vi "Add_Part_of_Track(101_and_11)-1.vi"(0 "[IN] Still connected\ntracks in group":T2, 1 "[IN] i for Probl\nem  Point Index":i32, 2 "[IN] i for # of Track \nwith Problem Point":i32, 3 "[IN] Minimal Sub\ntrack Length":i32, 7 "[IN] Subtrack":T1, 9 "[IN] Index in subtrack":i32, 11 "error IN":errorcluster, 12 "[IN] Index of problem\npoint inside subtrack":i32, 13 "[IN] # of subtrack conta\nining problem point":i32) -> (8 "[OUT] Subtrack":T1, 10 "[OUT] Last point in subtrack":i32, 15 "error OUT":errorcluster)   [LabVIEW 2013]
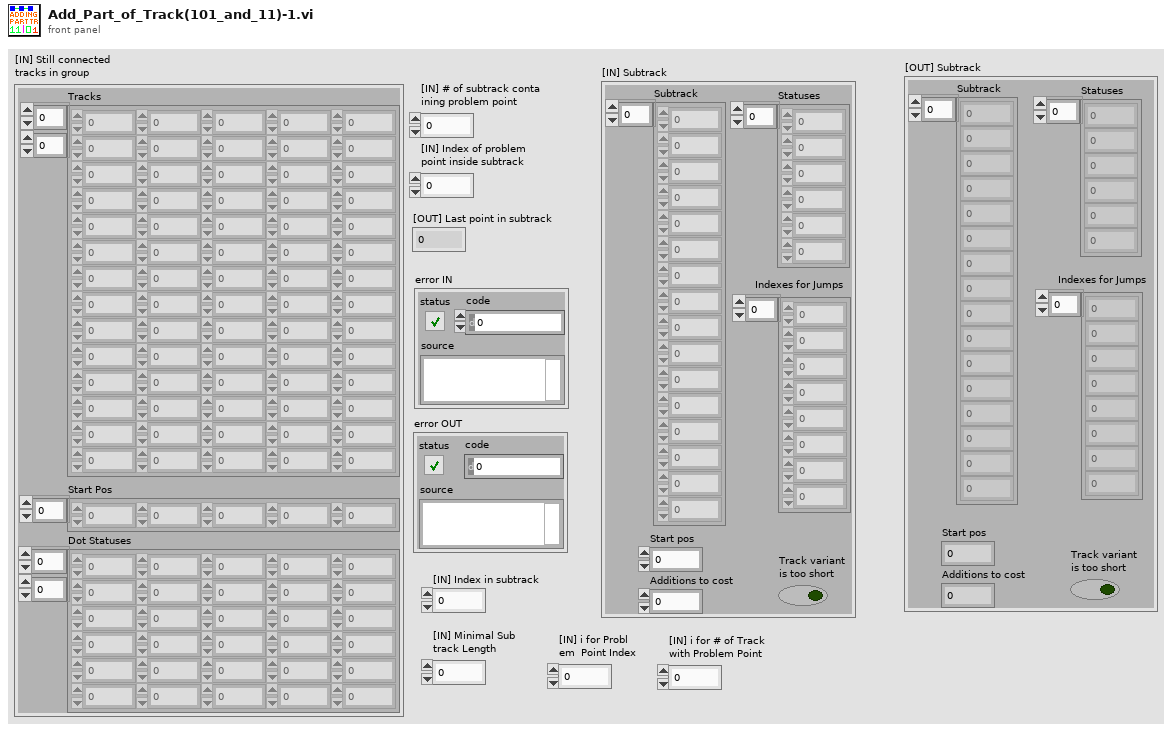
[diagram p1: front panel]
types:
  T1 = cluster{"Subtrack":dbl[], "Statuses":i16[], "Start pos":i32, "Additions to cost":i32, "Track variant \nis too short":bool, "Indexes for Jumps":i32[]}
  T2 = cluster{"Tracks":dbl[][], "Start Pos":i32[], "Dot Statuses":i16[][]}
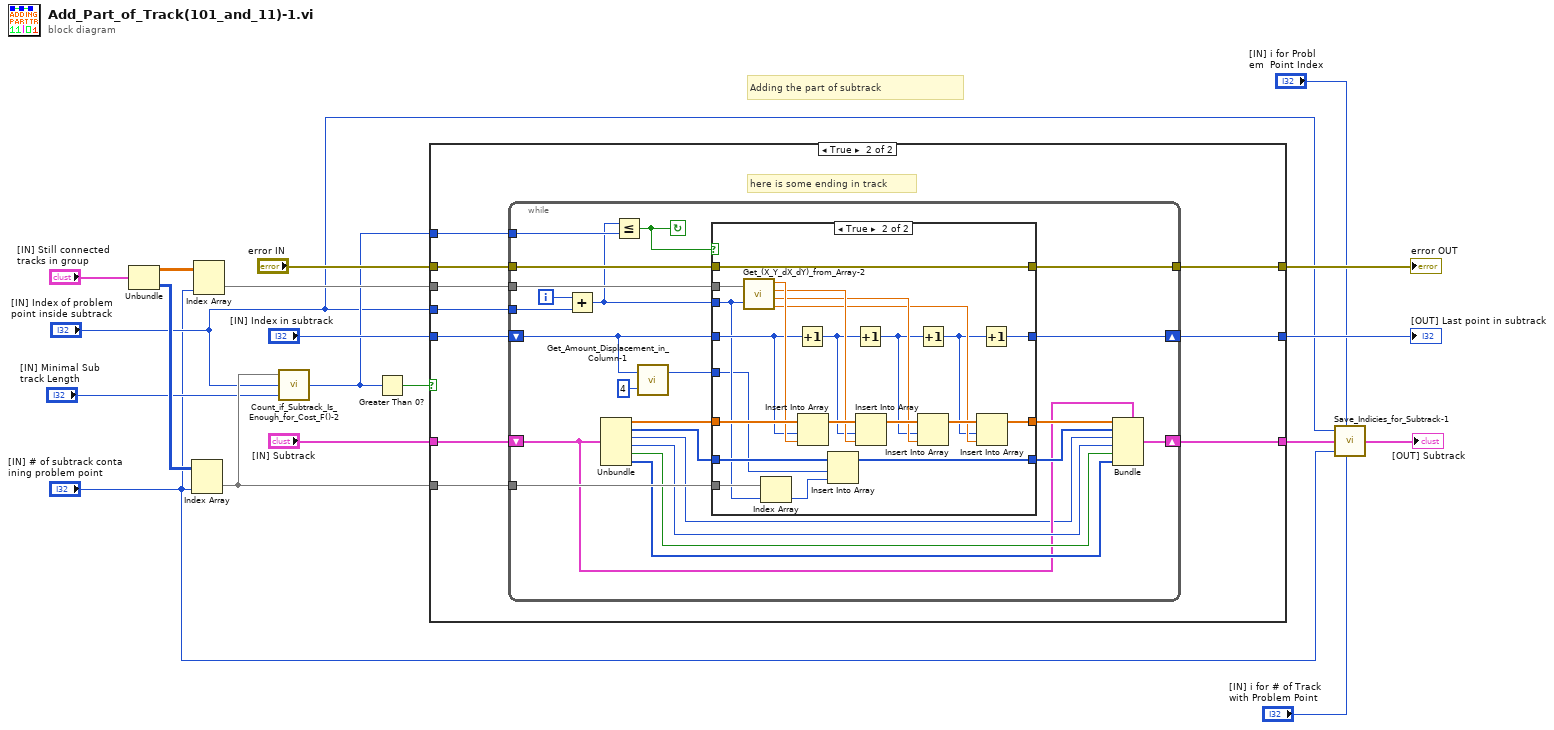
[diagram p0: block diagram]
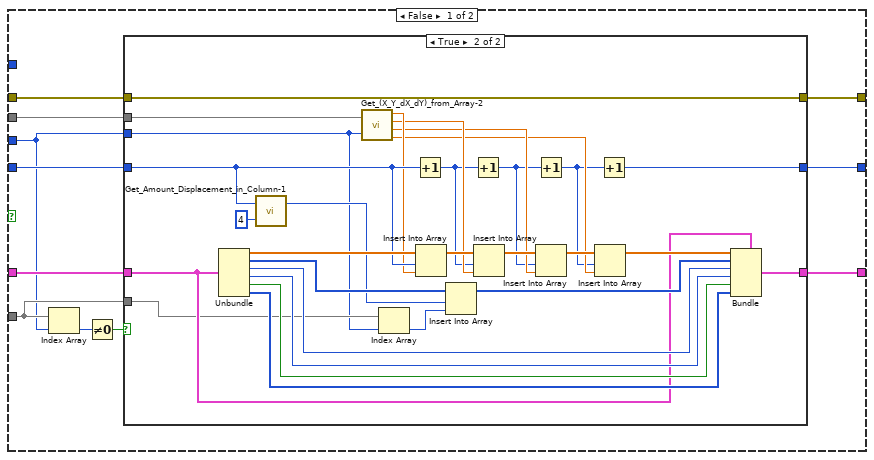
[diagram p2: hidden frame]
diagram:
  # "Adding the part of subtrack"
  n1 = Unbundle("[IN] Still connected\ntracks in group") -> ("Tracks"=w17:dbl[][], "Dot Statuses"=w15:i16[][])  [unwired: 1 out]
  n2 = Index Array(array=w15, index (col)="[IN] # of subtrack conta\nining problem point") -> (element=w8:i16[])  [unwired: 1 in]
  n3 = Index Array(array=w17, index (col)="[IN] # of subtrack conta\nining problem point") -> (element=w16:dbl[])  [unwired: 1 in]
  n4 = call "Count_if_Subtrack_Is_Enough_for_Cost_F()-2.vi"("[IN] Minimal Subtrack Length \n(Points without problems) for\nMaking Desicion"="[IN] Minimal Sub\ntrack Length", "[IN] Index of Problem \nPoint Inside Track"="[IN] Index of problem\npoint inside subtrack", "[IN] Dot Statuses in Track"=w8) -> ("[OUT] Index of Last \nPoint in Track"=w9:i32)  [unwired: 1 in, 1 out]
  n5 = Greater Than 0?(x=w9) -> (x > 0?=w10:bool)
  n6 = case shown="True" w10 {
    tunnel: "error IN" -> [w23 w72]
    tunnel: w16 -> [w22 w71]
    tunnel: [w25 w70] -> w14
    tunnel: [w20 w69] -> w13
    tunnel: "[IN] Subtrack" -> [w28 w68]
    tunnel: "[IN] Index in subtrack" -> [w27 w67]
    tunnel: w8 -> [w24 w66]
    tunnel: w9 -> [_ w65]
    tunnel: "[IN] Index of problem\npoint inside subtrack" -> [w21 w64]
    tunnel: [w26 w63] -> w6
    frame False {
      n7 = Index Array(array=w24, index=w21) -> (element=w30:i16)
      n8 = Not Equal To 0?(x=w30) -> (x != 0?=w29:bool)
      n9 = case shown="True" w29 {
        tunnel: w28 -> [w31 w52]
        tunnel: w27 -> [w32 w51]
        tunnel: [w31 w50] -> w26
        tunnel: [w32 w49] -> w25
        tunnel: w24 -> [_ w48]
        tunnel: w23 -> [w33 w34]
        tunnel: w22 -> [_ w47]
        tunnel: w21 -> [_ w46]
        tunnel: [w33 w34] -> w20
        frame False {
        }
        frame True {
          n10 = Unbundle(w52) -> ("Subtrack"=w62:dbl[], "Statuses"=w61:i16[], "Start pos"=w53:i32, "Additions to cost"=w58:i32, "Track variant \nis too short"=w57:bool, "Indexes for Jumps"=w56:i32[])
          n11 = call "Get_Amount_Displacement_in_Column-1.vi"("multiplier"=4, "# Rows"=w51) -> ("Displ amount"=w54:i32)  [unwired: 1 out]
          n12 = call "Get_(X_Y_dX_dY)_from_Array-2.vi"("(X,Y,dX,dY)"=w47, "Index of Displacement"=w46) -> ("X"=w45:dbl, "Y"=w43:dbl, "dX"=w40:dbl, "dY"=w37:dbl)
          n13 = Index Array(array=w48, index=w46) -> (element=w36:i16)
          n14 = Increment(x=w51) -> (x+1=w41:i32)
          n15 = Insert Into Array(array=w62, index=w51, new element=w45) -> (w44:dbl[])
          n16 = Insert Into Array(array=w61, index=w54, new element=w36) -> (w59:i16[])
          n17 = Increment(x=w41) -> (x+1=w39:i32)
          n18 = Insert Into Array(array=w44, index=w41, new element=w43) -> (w42:dbl[])
          n19 = Increment(x=w39) -> (x+1=w35:i32)
          n20 = Insert Into Array(array=w42, index=w39, new element=w40) -> (w38:dbl[])
          n21 = Insert Into Array(array=w38, index=w35, new element=w37) -> (w60:dbl[])
          n22 = Increment(x=w35) -> (x+1=w49:i32)
          n23 = Bundle(cluster=w52, "Subtrack"=w60, "Statuses"=w59, "Start pos"=w53, "Additions to cost"=w58, "Track variant \nis too short"=w57, "Indexes for Jumps"=w56) -> (w50:T1)
        }
      }
    }
    frame True {
      # "here is some ending in track"
      n24 = while {
        tunnel: w71 -> [w95]
        tunnel: w66 -> [w91]
        shift-right: [w88] -> w63
        shift-left: w68 -> [w82]
        tunnel: w72 -> [w84]
        tunnel: [w83] -> w69
        shift-right: [w81] -> w70
        shift-left: w67 -> [w79]
        tunnel: w65 -> [w76]
        tunnel: w64 -> [w73]
        i -> [w75]
        stop <- w93 continue-if-true
        n25 = Add(x=w75, y=w73) -> (x+y=w74:i32)
        n26 = Unbundle(w82) -> ("Subtrack"=w94:dbl[], "Statuses"=w92:i16[], "Start pos"=w77:i32, "Additions to cost"=w87:i32, "Track variant \nis too short"=w86:bool, "Indexes for Jumps"=w85:i32[])
        n27 = Less Or Equal?(x=w74, y=w76) -> (x <= y?=w93:bool)
        n28 = call "Get_Amount_Displacement_in_Column-1.vi"("multiplier"=4, "# Rows"=w79) -> ("Displ amount"=w78:i32)  [unwired: 1 out]
        n29 = case shown="True" w93 {
          tunnel: w95 -> [_ w121]
          tunnel: w94 -> [w98 w120]
          tunnel: w79 -> [w96 w118]
          tunnel: w74 -> [_ w107]
          tunnel: w92 -> [w99 w109]
          tunnel: w91 -> [_ w108]
          tunnel: [w98 w105] -> w90
          tunnel: [w99 w104] -> w89
          tunnel: w84 -> [w97 w103]
          tunnel: [w97 w103] -> w83
          tunnel: [w96 w100] -> w81
          tunnel: w78 -> [_ w102]
          frame False {
          }
          frame True {
            n30 = call "Get_(X_Y_dX_dY)_from_Array-2.vi"("(X,Y,dX,dY)"=w121, "Index of Displacement"=w107) -> ("X"=w119:dbl, "Y"=w116:dbl, "dX"=w113:dbl, "dY"=w110:dbl)
            n31 = Index Array(array=w108, index=w107) -> (element=w106:i16)
            n32 = Increment(x=w118) -> (x+1=w114:i32)
            n33 = Insert Into Array(array=w120, index=w118, new element=w119) -> (w117:dbl[])
            n34 = Insert Into Array(array=w109, index=w102, new element=w106) -> (w104:i16[])
            n35 = Increment(x=w114) -> (x+1=w112:i32)
            n36 = Insert Into Array(array=w117, index=w114, new element=w116) -> (w115:dbl[])
            n37 = Increment(x=w112) -> (x+1=w101:i32)
            n38 = Insert Into Array(array=w115, index=w112, new element=w113) -> (w111:dbl[])
            n39 = Insert Into Array(array=w111, index=w101, new element=w110) -> (w105:dbl[])
            n40 = Increment(x=w101) -> (x+1=w100:i32)
          }
        }
        n41 = Bundle(cluster=w82, "Subtrack"=w90, "Statuses"=w89, "Start pos"=w77, "Additions to cost"=w87, "Track variant \nis too short"=w86, "Indexes for Jumps"=w85) -> (w88:T1)
      }
    }
  }
  "[OUT] Last point in subtrack" <- w14
  "error OUT" <- w13
  n42 = call "Save_Indicies_for_Subtrack-1.vi"("[IN] Index of Origin/Problem \nPoint inside Original Track (X1)"="[IN] Index of problem\npoint inside subtrack", "[IN] i for X1"="[IN] i for Probl\nem  Point Index", "[IN] Subtrack"=w6, "[IN] Index of Track Conta-\nining Origin/Problem (X2)"="[IN] # of subtrack conta\nining problem point", "[IN] i for X2"="[IN] i for # of Track \nwith Problem Point") -> ("[OUT] Subtrack"=→"[OUT] Subtrack":T1)
